vi "Frame decomposition.vi"() -> ()   [LabVIEW 2020]
uses:
  <vilib>/xnet/xnet.llb/XNET Frame CAN.ctl
  <vilib>/xnet/xnet.llb/XNET Frame Type CAN.ctl
  <resource>/objmgr/xnet.rc
panel:
  out "XNET Frame":refnum<k21>
  out "Frames":refnum<k21>[](array[refnum])
  out "Payload Length":u32
  out "Identifier":u32
  out "Name (Short)":string
  out "CAN frame":T1 {"payload" format="%x"; "timestamp" format="%<%.7X\n%x>T"; "type" items=["CAN Data"=0, "CAN Remote"=1, "CAN Bus Error"=2, "CAN 2.0 Data"=8, "CAN FD Data"=16, "CAN FD+BRS Data"=24, "J1939 Data"=192, "Delay"=224, "Log Trigger"=225, "Start Trigger"=226]; "identifier" format="%08x"}
  out "Frame":refnum<k21>
  out "Number of Bits":u32
  out "Data Type":u32(ring) items=["Signed", "Unsigned", "IEEE Float", "Byte Array"]
  out "Unit":string
  out "Start Bit":u32
  out "Scaling Offset":dbl
  out "Scaling Factor":dbl
  out "XNET Signal":refnum<k21>
  in  "Numeric":dbl
  out "Signals":refnum<k21>[](array[refnum])
  out "frame list out":refnum<k21>[](array[refnum])
  out "Data Array":T1[](array[typedef]) {"payload" format="%x"; "timestamp" format="%<%.7X\n%x>T"; "type" items=["CAN Data"=0, "CAN Remote"=1, "CAN Bus Error"=2, "CAN 2.0 Data"=8, "CAN FD Data"=16, "CAN FD+BRS Data"=24, "J1939 Data"=192, "Delay"=224, "Log Trigger"=225, "Start Trigger"=226]; "identifier" format="%08x"}
  in  "cluster (:memory:)":refnum<k21>=":memory:"
  out "number":u8 format="%.0x"
  in  "Array":bool[](array[boolean])
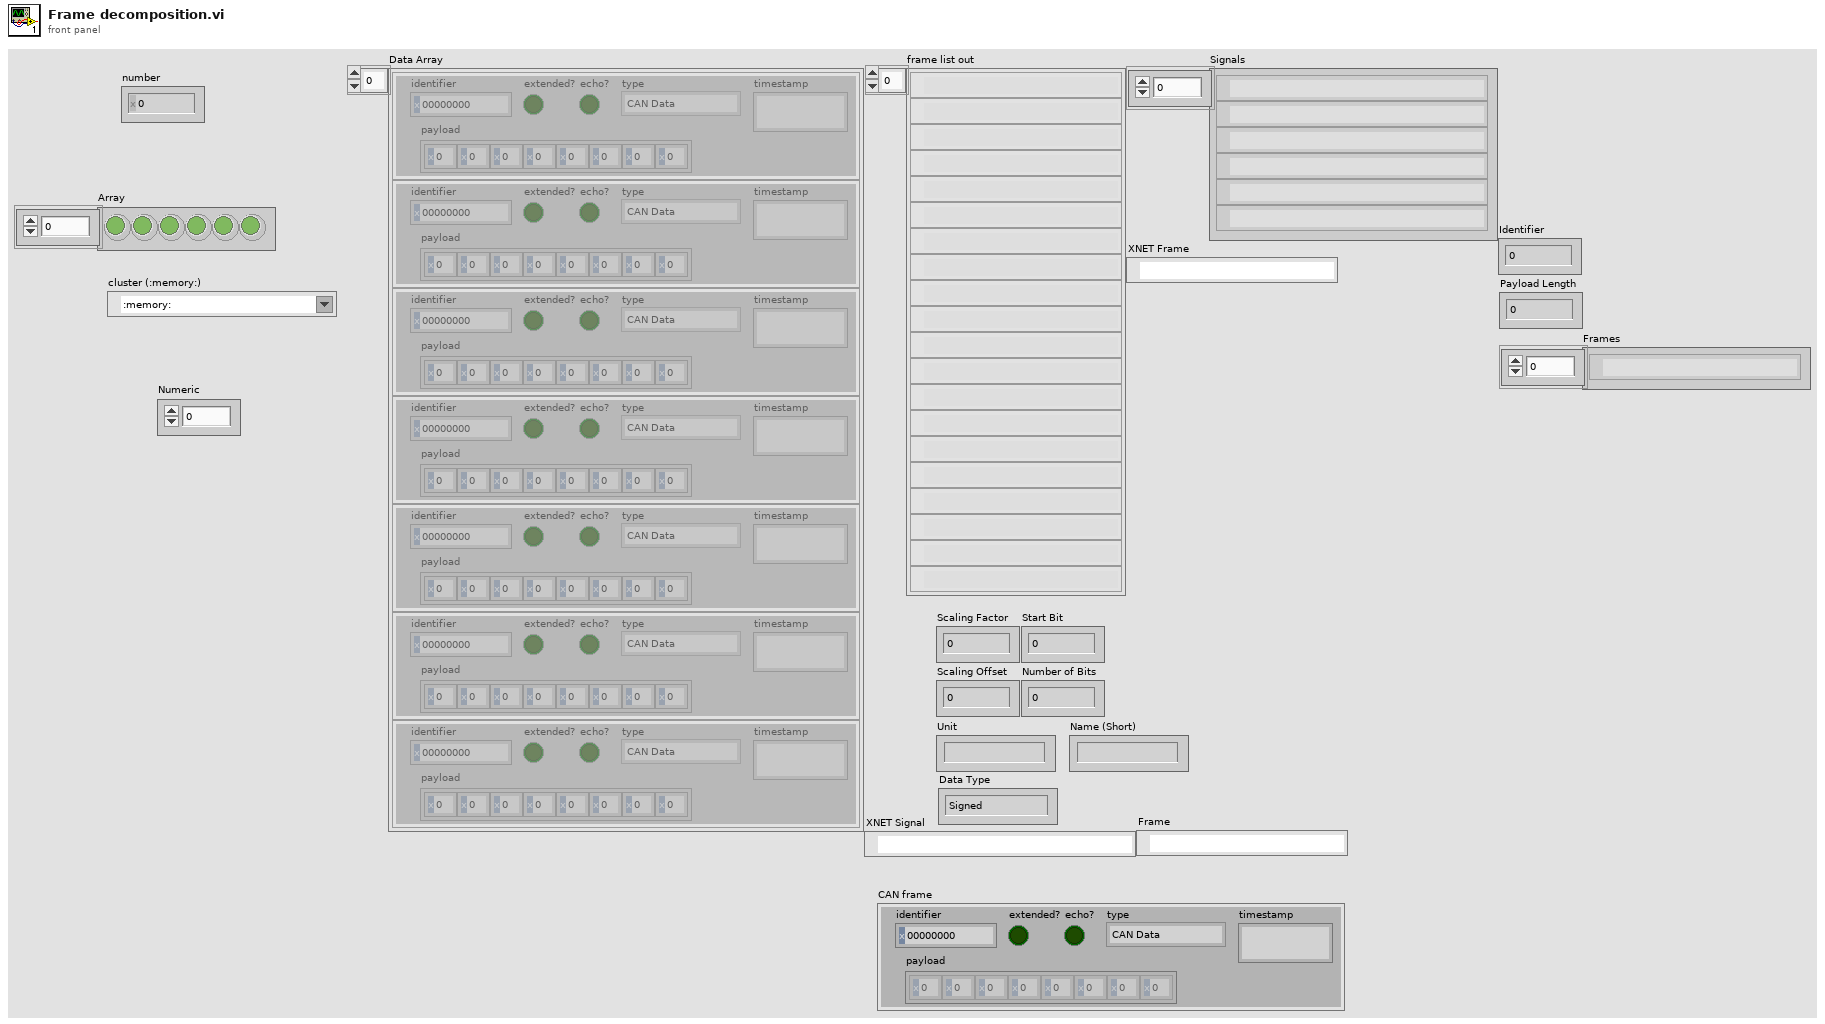
[diagram p1: front panel]
types:
  T1 = typedef "XNET Frame CAN.ctl" = cluster{"timestamp":timestamp, "payload":u8[], "identifier":u32, "type":T2, "extended?":bool, "echo?":bool}
  T2 = typedef "XNET Frame Type CAN.ctl" = u8
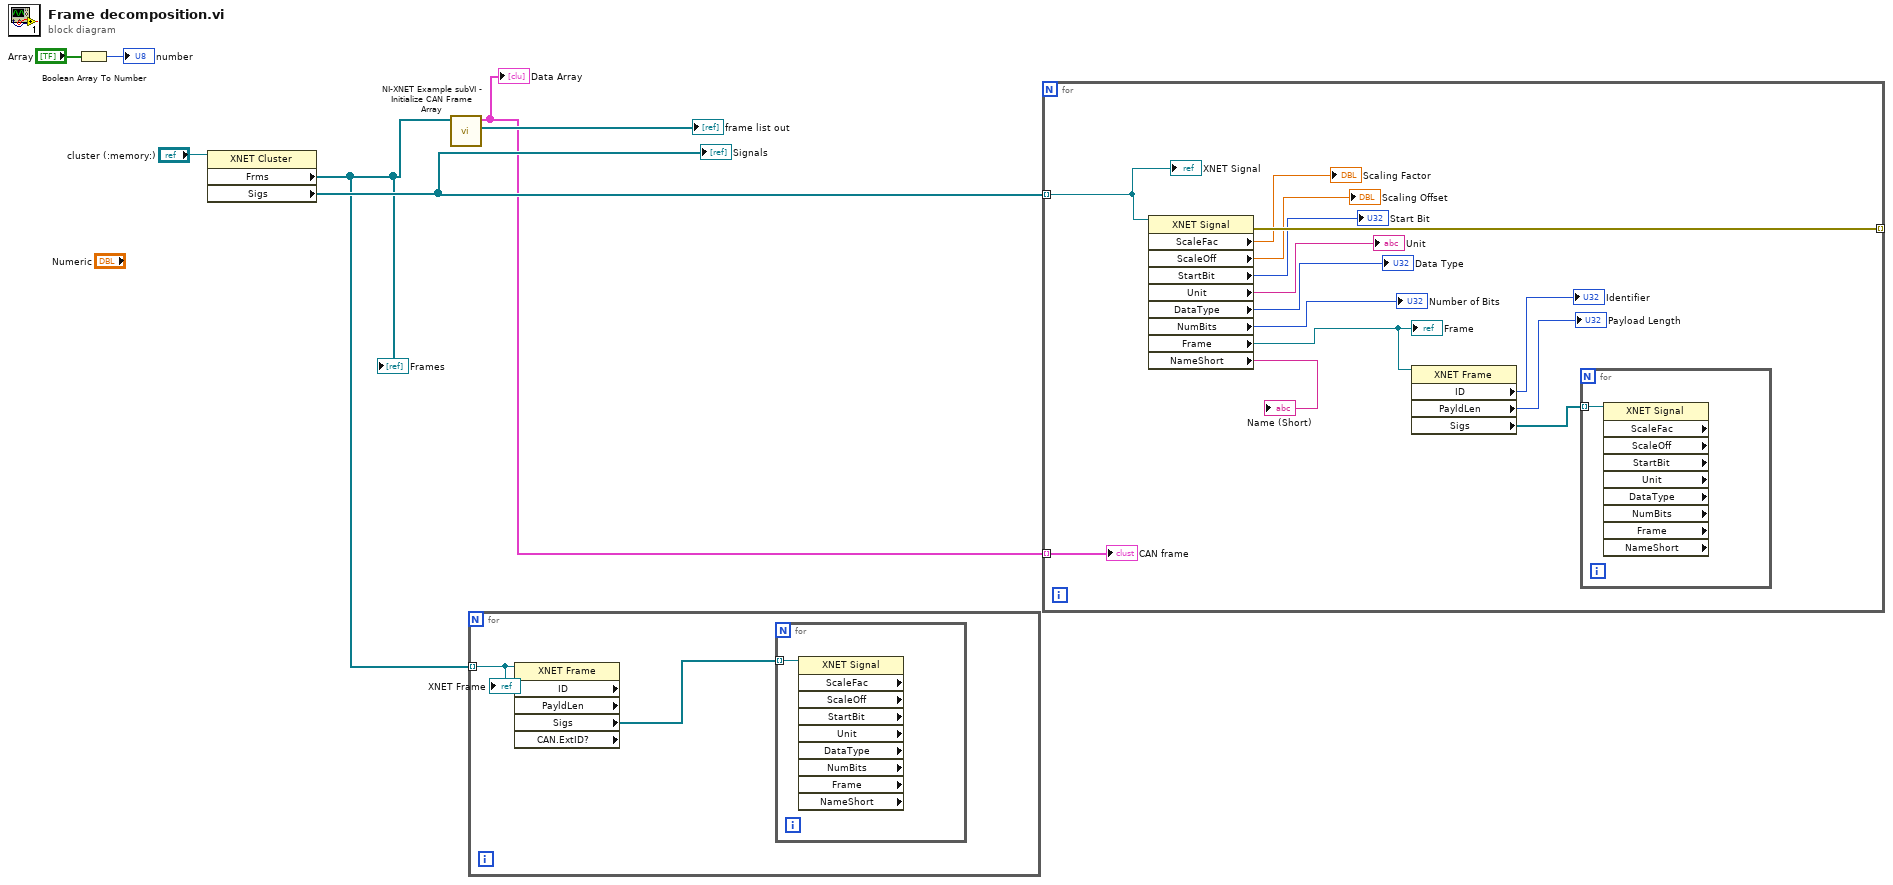
[diagram p0: block diagram]
diagram:
  n1 = Boolean Array To Number(Boolean array="Array") -> (number=→"number":u32)
  n2 = property class="XNET Cluster"(reference="cluster (:memory:)") -> ("Frms"=w2:refnum<k21>[], "Sigs"=w4:refnum<k21>[])  [unwired: 1 in, 2 out]
  "Signals" <- w4
  "Frames" <- w2
  n3 = call "NI-XNET Example subVI - Initialize CAN Frame Array.vi"("frame list in"=w2) -> ("frame list out"=→"frame list out":refnum<k21>[], "Data Array"=w3:T1[])  [unwired: 1 in, 6 out]
  "Data Array" <- w3
  n4 = for {
    tunnel: w2 -> [w8] mode=indexing
    n5 = property class="XNET Frame" props=["ID", "PayldLen", "Sigs", "CAN.ExtID?"](reference=w8) -> ("Sigs"=w9:refnum<k21>[])  [unwired: 1 in, 5 out]
    n6 = for {
      tunnel: w9 -> [w10] mode=indexing
      n7 = property class="XNET Signal" props=["ScaleFac", "ScaleOff", "StartBit", "Unit", "DataType", "NumBits", "Frame", "NameShort"](reference=w10) -> ()  [unwired: 1 in, 10 out]
    }
    "XNET Frame" <- w8
  }
  n8 = for {
    tunnel: w4 -> [w24] mode=indexing
    tunnel: [w23] -> _ mode=indexing
    tunnel: w3 -> [w16] mode=indexing
    n9 = property class="XNET Signal"(reference=w24) -> (error out=w23:errorcluster, "ScaleFac"=→"Scaling Factor":dbl, "ScaleOff"=→"Scaling Offset":dbl, "StartBit"=→"Start Bit":u32, "Unit"=→"Unit":string, "DataType"=→"Data Type":u32, "NumBits"=→"Number of Bits":u32, "Frame"=w14:refnum<k21>, "NameShort"=→"Name (Short)":string)  [unwired: 1 in, 1 out]
    "Frame" <- w14
    n10 = property class="XNET Frame"(reference=w14) -> ("ID"=→"Identifier":u32, "PayldLen"=→"Payload Length":u32, "Sigs"=w11:refnum<k21>[])  [unwired: 1 in, 2 out]
    n11 = for {
      tunnel: w11 -> [w25] mode=indexing
      n12 = property class="XNET Signal" props=["ScaleFac", "ScaleOff", "StartBit", "Unit", "DataType", "NumBits", "Frame", "NameShort"](reference=w25) -> ()  [unwired: 1 in, 10 out]
    }
    "XNET Signal" <- w24
    "CAN frame" <- w16
  }
